vi "gyro_horizon.vi"(5 "center":cluster{"x":i32, "y":i32}={"x"=105, "y"=32}, 6 "stabile":bool=TRUE, 7 "size":i32(slide)=29 scale=0.0..100.0, 9 "rotate":cluster{"pitch":i32, "roll":i32, "yaw":i32}={"pitch"=-95, "roll"=-49, "yaw"=27} {"pitch" scale=-180.0..180.0; "roll" scale=-180.0..180.0; "yaw" scale=-180.0..180.0}, 11 "pict in":picture) -> (3 "gyro_horizon":picture)   [LabVIEW 2011]
uses:
  <vilib>/Analysis/baseanly.llb/Real A x B.vi
  <vilib>/Analysis/NI_AALBase.lvlib
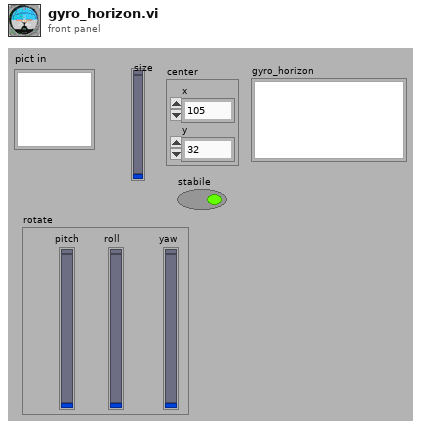
[diagram p1: front panel]
types:
  T1 = typedef "NI_Matrix.lvlib/RealMatrix.ctl" = dbl[][]
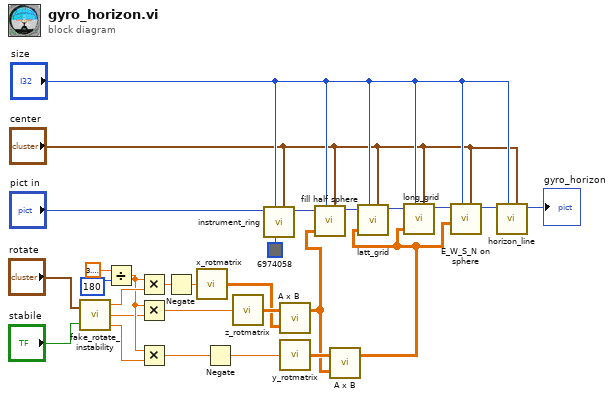
[diagram p0: block diagram]
diagram:
  n1 = call "fake_rotate_instability.vi"("rotation"="rotate", "stabile"="stabile") -> ("Pitch"=w25:dbl, "Roll"=w23:dbl, "Yow"=w22:dbl)
  n2 = Divide(x=3.141592653589793, y=180) -> (x/y=w24:dbl)
  n3 = Multiply(x=w24, y=w25) -> (x*y=w19:dbl)
  n4 = Multiply(x=w24, y=w23) -> (x*y=w17:dbl)
  n5 = Multiply(x=w24, y=w22) -> (x*y=w18:dbl)
  n6 = Negate(x=w19) -> (-x=w6:dbl)
  n7 = call "x_rotmatrix.vi"("x-angle"=w6) -> ("x-matrix"=w4:dbl[][])
  n8 = Negate(x=w18) -> (-x=w7:dbl)
  n9 = call "z_rotmatrix.vi"("z-angle"=w17) -> ("z-matrix"=w5:dbl[][])
  n10 = call "instrument_ring.vi"("center"="center", "inside color"=u32 6974058, "size"="size", "pict in"="pict in") -> ("new picture"=w14:picture)  [unwired: 6 in]
  n11 = call-poly <vilib>:"A x B.vi"("B"=w4, "A"=w5) -> ("A x B"=w1:T1)  [unwired: 1 out]
  n12 = call "y_rotmatrix.vi"("y-angle"=w7) -> ("y-matrix"=w16:dbl[][])
  n13 = call "fill half sphere.vi"("pict in"=w14, "size"="size", "v-matrix"=w1, "center"="center") -> ("pict out"=w15:picture)  [unwired: 6 in]
  n14 = call-poly <vilib>:"A x B.vi"("B"=w1, "A"=w16) -> ("A x B"=w2:T1)  [unwired: 1 out]
  n15 = call "latt_grid.vi"("pict in"=w15, "size"="size", "rotation"=w2, "center"="center") -> ("pict out"=w28:picture)  [unwired: 6 in]
  n16 = call "long_grid.vi"("pict in"=w28, "size"="size", "rotation"=w2, "center"="center") -> ("pict out"=w13:picture)  [unwired: 6 in]
  n17 = call "E_W_S_N on sphere.vi"("center"="center", "size"="size", "rotation"=w2, "pict in"=w13) -> ("pict out"=w11:picture)  [unwired: 5 in]
  n18 = call "horizon_line.vi"("center"="center", "size"="size", "pict in"=w11) -> ("new out"=→"gyro_horizon":picture)  [unwired: 7 in]
